vi "Begin.vi"(8 "error in":errorcluster) -> (0 "error out":errorcluster)   [LabVIEW 2023]
doc: "Called before other user functions, this VI can be used to open I/O refnums, load in file data, and do general program initialization. Notice that the <B>error out</B> terminal is simply used for data flow. Wiring it to other structures or subVIs ensures that this VI runs first."
uses:
  <vilib>/Rock Robotics/WPI/DriverStation/WPI_DriverStationRobotMode2.ctl
  <vilib>/Rock Robotics/WPI/Joystick/WPI_JoystickDeviceEnum.ctl
  Swerve/Implementation/Swerve Setpoints2.ctl
  Swerve/Implementation/Swerve Operations.ctl
  <vilib>/Rock Robotics/SystemInterfaces/DIO/FPGA_DIOChannel.ctl
  <vilib>/Rock Robotics/WPI/Solenoid/WPI_SolenoidChannel.ctl
  <vilib>/Rock Robotics/WPI/Solenoid/WPI_SolenoidValue.ctl
  <vilib>/Rock Robotics/WPI/SafetyOutput/WPI_SafetyOutputConfigMenu.ctl
  <vilib>/Rock Robotics/WPI/ThirdParty/REV Robotics/REVLib/Typedef/Spark MAX Idle Mode.ctl
  <vilib>/Rock Robotics/WPI/ThirdParty/REV Robotics/REVLib/Typedef/Spark MAX Sensor Type.ctl
  <vilib>/Rock Robotics/WPI/ThirdParty/REV Robotics/REVLib/Typedef/Spark MAX Control Type.ctl
  Robot Global Data.vi
  <vilib>/Rock Robotics/Network Tables/NT Write String Array.vi
  <vilib>/Rock Robotics/WPI/Solenoid/WPI_SolenoidOpenDouble.vi
  <vilib>/Rock Robotics/WPI/Solenoid/WPI_SolenoidSetEnum.vi
  <vilib>/Rock Robotics/WPI/Utilities/WPI_GetSetVariantRefNum.vi
  <vilib>/Rock Robotics/SystemInterfaces/DIO/FPGA_DIOPWMChannel.ctl
  Arm/Implementation/Arm Setpoints.ctl
panel:
  in  "Swerve PID":T1={"P Gain"=1.1, "I Gain"=0.0, "D Gain"=0.0, "F Gain"=0.0, "I Zone"=0.0, "Min Output"=-1.0, "Max Output"=1.0}
  in  "PID Constants 2":T1={"P Gain"=2.0, "I Gain"=0.0, "D Gain"=0.0, "F Gain"=0.0, "I Zone"=0.0, "Min Output"=-1.0, "Max Output"=1.0}
  in  "PID Constants":T1={"P Gain"=0.8, "I Gain"=0.0, "D Gain"=0.0, "F Gain"=0.0, "I Zone"=0.0, "Min Output"=-1.0, "Max Output"=1.0}
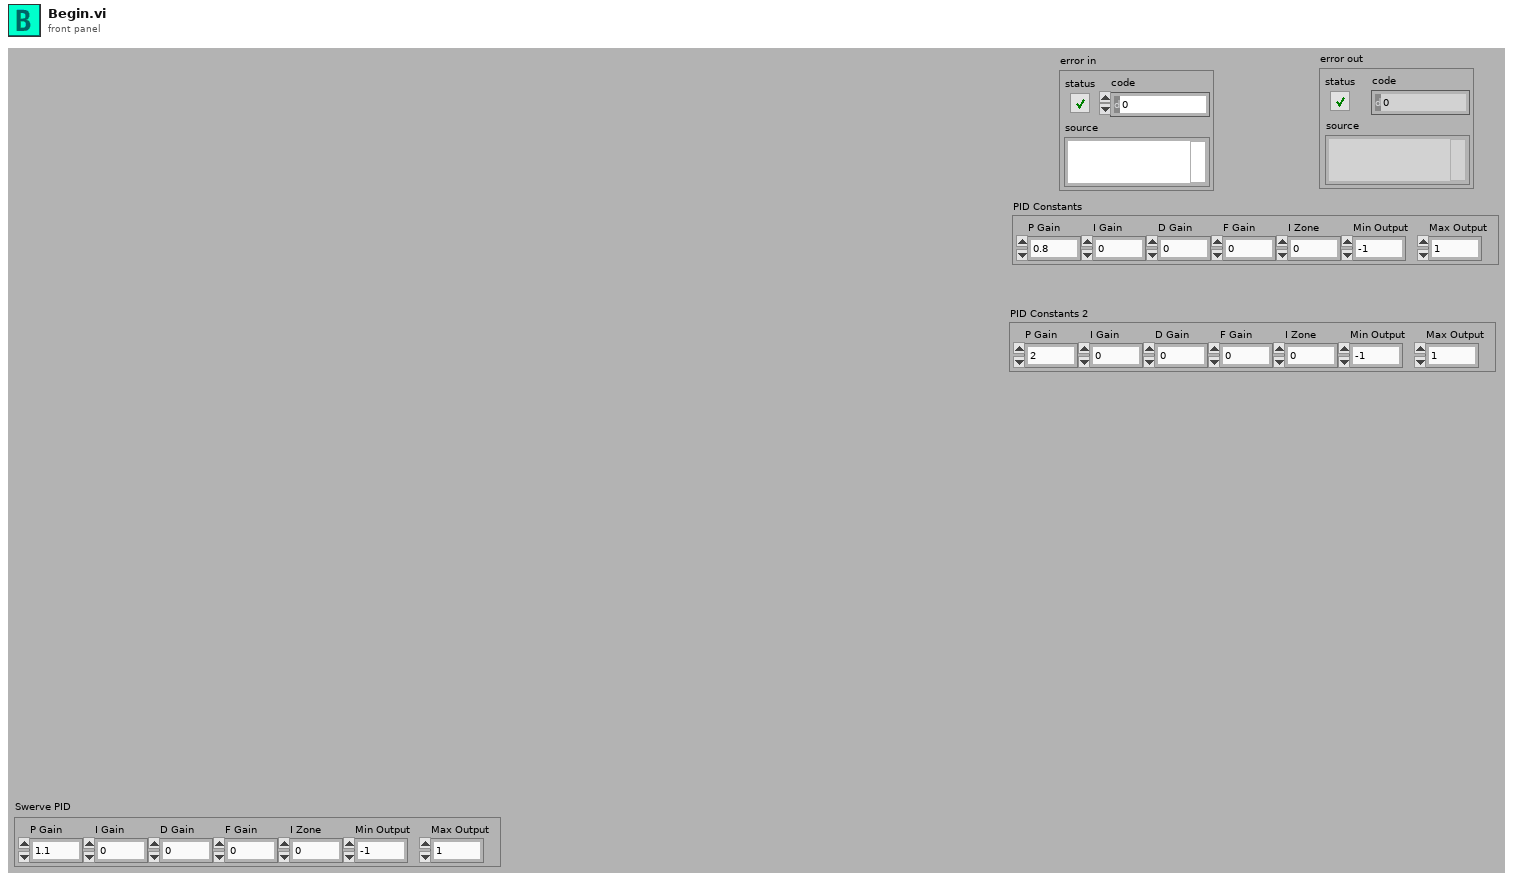
[diagram p1: front panel]
types:
  T1 = cluster{"P Gain":dbl, "I Gain":dbl, "D Gain":dbl, "F Gain":dbl, "I Zone":dbl, "Min Output":dbl, "Max Output":dbl}
  T2 = typedef "FPGA_DIOChannel.ctl" = enum8{"DIO 0", "DIO 1", "DIO 2", "DIO 3", "DIO 4", "DIO 5", "DIO 6", "DIO 7", "DIO 8", "DIO 9", "DIO MXP 0", "DIO MXP 1", "DIO MXP 2", "DIO MXP 3", "DIO MXP 4", "DIO MXP 5", "DIO MXP 6", "DIO MXP 7", "DIO MXP 8", "DIO MXP 9", "DIO MXP 10", "DIO MXP 11", "DIO MXP 12", "DIO MXP 13", "DIO MXP 14", "DIO MXP 15", "SPI Port CS1", "SPI Port CS2", "SPI Port CS3", "SPI Port MISO", "SPI Port MOSI", "Invalid"}
  T3 = typedef "Swerve Setpoints2.ctl" = cluster{"Operation":T4, "Gyro":dbl, "FWD":dbl, "STR":dbl, "X rotate":dbl, "Y rotate":dbl, "Time":dbl, "Distance":dbl, "Right Trigger":dbl, "Angle":dbl, "Start Angle":dbl, "Tag ID":dbl, "Start Positions":dbl[]}
  T4 = typedef "Swerve Operations.ctl" = enum16{"Reserve", "Read Current", "Immediate", "Stop", "Balance", "Direct  Joystick Drive", "Joystick Drive", "Drive for Distance", "Drive for Time", "Turn to Angle", "Drive to Angle(Time)", "Drive to Angle(Distance)", "Look At Cone", "Look At Cube", "Move To Tape", "Move To Tag"}
  T5 = typedef "WPI_JoystickDeviceEnum.ctl" = enum16{"USB 0", "USB 1", "USB 2", "USB 3", "USB 4", "USB 5"}
  T6 = typedef "WPI_DriverStationRobotMode2.ctl" = enum16{"Autonomous Disabled", "Autonomous Enabled", "Teleop Disabled", "Teleop Enabled", "Disconnected", "Finish", "Test Disabled", "Test Enabled", "Emergency Stopped"}
  T7 = typedef "Spark MAX Sensor Type.ctl" = enum16{"No Sensor", "Hall Sensor", "Encoder", "-Not Available-", "Analog", "Alternate Encoder", "Duty Cycle"}
  T8 = typedef "Spark MAX Idle Mode.ctl" = enum16{"Coast", "Brake"}
  T9 = typedef "WPI_SafetyOutputConfigMenu.ctl" = enum16{"Enable", "Disable"}
  T10 = typedef "WPI_MotorControlDeviceRef.ctl" = cluster{"DeviceStatus":errorcluster, "Type":T11, "PWM":cluster{"PWM Channel":T12, "DeadBand":T13}, "CAN":cluster{"Device Number":u8, "SetOutput VI Ref":variant, "GetOutput VI Ref":variant, "Enable VI Ref":variant, "Disable VI Ref":variant, "Data":variant}, "Invert":bool, "DIO PWM":cluster{"PWM \"Enable\" Channel":T12, "DIOChannel":T2, "PWM Rate":dbl}}
  T11 = typedef "WPI_MotorControlType.ctl" = enum16{"PWM", "CAN", "DIO PWM"}
  T12 = typedef "FPGA_DIOPWMChannel.ctl" = enum8{"PWM 0", "PWM 1", "PWM 2", "PWM 3", "PWM 4", "PWM 5", "PWM 6", "PWM 7", "PWM 8", "PWM 9", "PWM MXP 0", "PWM MXP 1", "PWM MXP 2", "PWM MXP 3", "PWM MXP 4", "PWM MXP 5", "PWM MXP 6", "PWM MXP 7", "PWM MXP 8", "PWM MXP 9", "Invalid"}
  T13 = typedef "WPI_PWMDeadband.ctl" = cluster{"Name":string, "maxPositivePwm":i32, "minPositivePwm":i32, "centerPwm":i32, "maxNegativePwm":i32, "minNegativePwm":i32, "angularRange":u16}
  T14 = typedef "WPI_JoystickDevRef.ctl" = cluster{"Device":T5}
  T15 = typedef "ADIS16470 Device Reference.ctl" = cluster{"DevStatus":errorcluster, "Hardware Config":T16, "Calibration Complete":refnum<notifier>, "Status Reference":refnum<data-value>, "Data Reference":refnum<data-value>, "Sychronous Process VI":T19, "Cmd FIFO":refnum<k33>, "Source":T20, "Data FIFO":refnum<k33>, "Calibration Time (ms)":u32, "Data Reference":refnum<data-value>}
  T16 = typedef "ADIS16470 Hardware Configuration.ctl" = cluster{"SPI Clock Rate (Hz)":dbl, "IMU SPI Mode (3)":T17, "IMU Reset Pin":T2, "IMU SPI Bus":T18, "IMU Data Ready Pin":T2, "Stall Config":cluster{"Pow2BytesPerRead":u8, "StallTicks":u16, "CsToSclkTicks":u8}}
  T17 = typedef "WPI_SPIMode.ctl" = enum16{"Mode 0 (Clk Idle Low,Sample on Leading)", "Mode 1 (Clk Idle Low,Sample on Trailing)", "Mode 2 (Clk Idle High,Sample on Leading)", "Mode 3 (Clk Idle High,Sample on Trailing)"}
  T18 = typedef "spi_bus.ctl" = enum16{"SPI On-Board, CS0", "SPI On-Board, CS1", "SPI On-Board, CS2", "SPI On-Board, CS3", "SPI MXP", "Invalid"}
  T19 = typedef "ADIS16470 Process.ctl" = refnum<vi>
  T20 = typedef "FPGA_CounterEncoderSourceConvertionLVSourceType.ctl" = cluster{"DevStatus":errorcluster, "AnalogTriggerMode?":bool, "DigitalMode":cluster{"DIO Channel":T21}, "AnalogTriggerMode":cluster{"AnalogTriggerIndex":T22, "OutputType":T23}}
  T21 = typedef "FPGA_DIODigitalSourceChannel.ctl" = enum8{"DIO 0", "DIO 1", "DIO 2", "DIO 3", "DIO 4", "DIO 5", "DIO 6", "DIO 7", "DIO 8", "DIO 9", "DIO MXP 0", "DIO MXP 1", "DIO MXP 2", "DIO MXP 3", "DIO MXP 4", "DIO MXP 5", "DIO MXP 6", "DIO MXP 7", "DIO MXP 8", "DIO MXP 9", "DIO MXP 10", "DIO MXP 11", "DIO MXP 12", "DIO MXP 13", "DIO MXP 14", "DIO MXP 15", "SPI Port CS1", "SPI Port CS2", "SPI Port CS3", "SPI Port MISO", "SPI Port MOSI", "Disabled"}
  T22 = typedef "FPGA_AnalogTriggerIndex.ctl" = enum8{"Trig 0", "Trig 1", "Trig 2", "Trig 3", "Trig 4", "Trig 5", "Trig 6", "Trig 7", "Invalid"}
  T23 = typedef "FPGA_AnalogTriggerOutType.ctl" = enum16{"InWindow", "TriggerState", "Rising", "Falling"}
  T24 = typedef "WPI_DigitalInputDevRef.ctl" = cluster{"DevStatus":errorcluster, "DIO Channel":T2}
  T25 = typedef "WPI_SolenoidValue.ctl" = enum16{"Off", "On", "Forward", "Reverse"}
  T26 = typedef "WPI_SolenoidChannel.ctl" = enum8{"Solenoid 0", "Solenoid 1", "Solenoid 2", "Solenoid 3", "Solenoid 4", "Solenoid 5", "Solenoid 6", "Solenoid 7", "Solenoid 8", "Solenoid 9", "Solenoid 10", "Solenoid 11", "Solenoid 12", "Solenoid 13", "Solenoid 14", "Solenoid 15", "Invalid"}
  T27 = typedef "WPI_CompressorDevRef.ctl" = cluster{"DevStatus":errorcluster, "Pneumatics Control Module":u8}
  T28 = typedef "WPI_SolenoidDevRef.ctl" = cluster{"DevStatus":errorcluster, "Pneumatics Control Module":u8, "Forward Solenoid Channel":T26, "Reverse Solenoid Channel":T26}
  T29 = typedef "WPI_PWMDeviceRef.ctl" = cluster{"DeviceStatus":errorcluster, "PWM Channel":T12}
  T30 = typedef "Spark MAX Control Type.ctl" = enum16{"Percent VBus", "Voltage", "Velocity", "Position", "Smart Motion", "Current", "Smart Velocity"}
  T31 = typedef "Arm Setpoints.ctl" = cluster{"Operation":enum16{"Reserve", "Read Current", "Immediate", "Move to position", "Adjust position", "Cube extend", "Cone extend", "Rotate Arm Joints", "Maintain Angle", "Retract", "Go_to_next"}, "X Position":dbl, "Y Position":dbl, "Up":dbl, "Right":dbl, "Joint 1 Angle":dbl[], "Joint 2 Angle":dbl[], "Joint 1 Speed":dbl, "Joint 2 Speed":dbl}
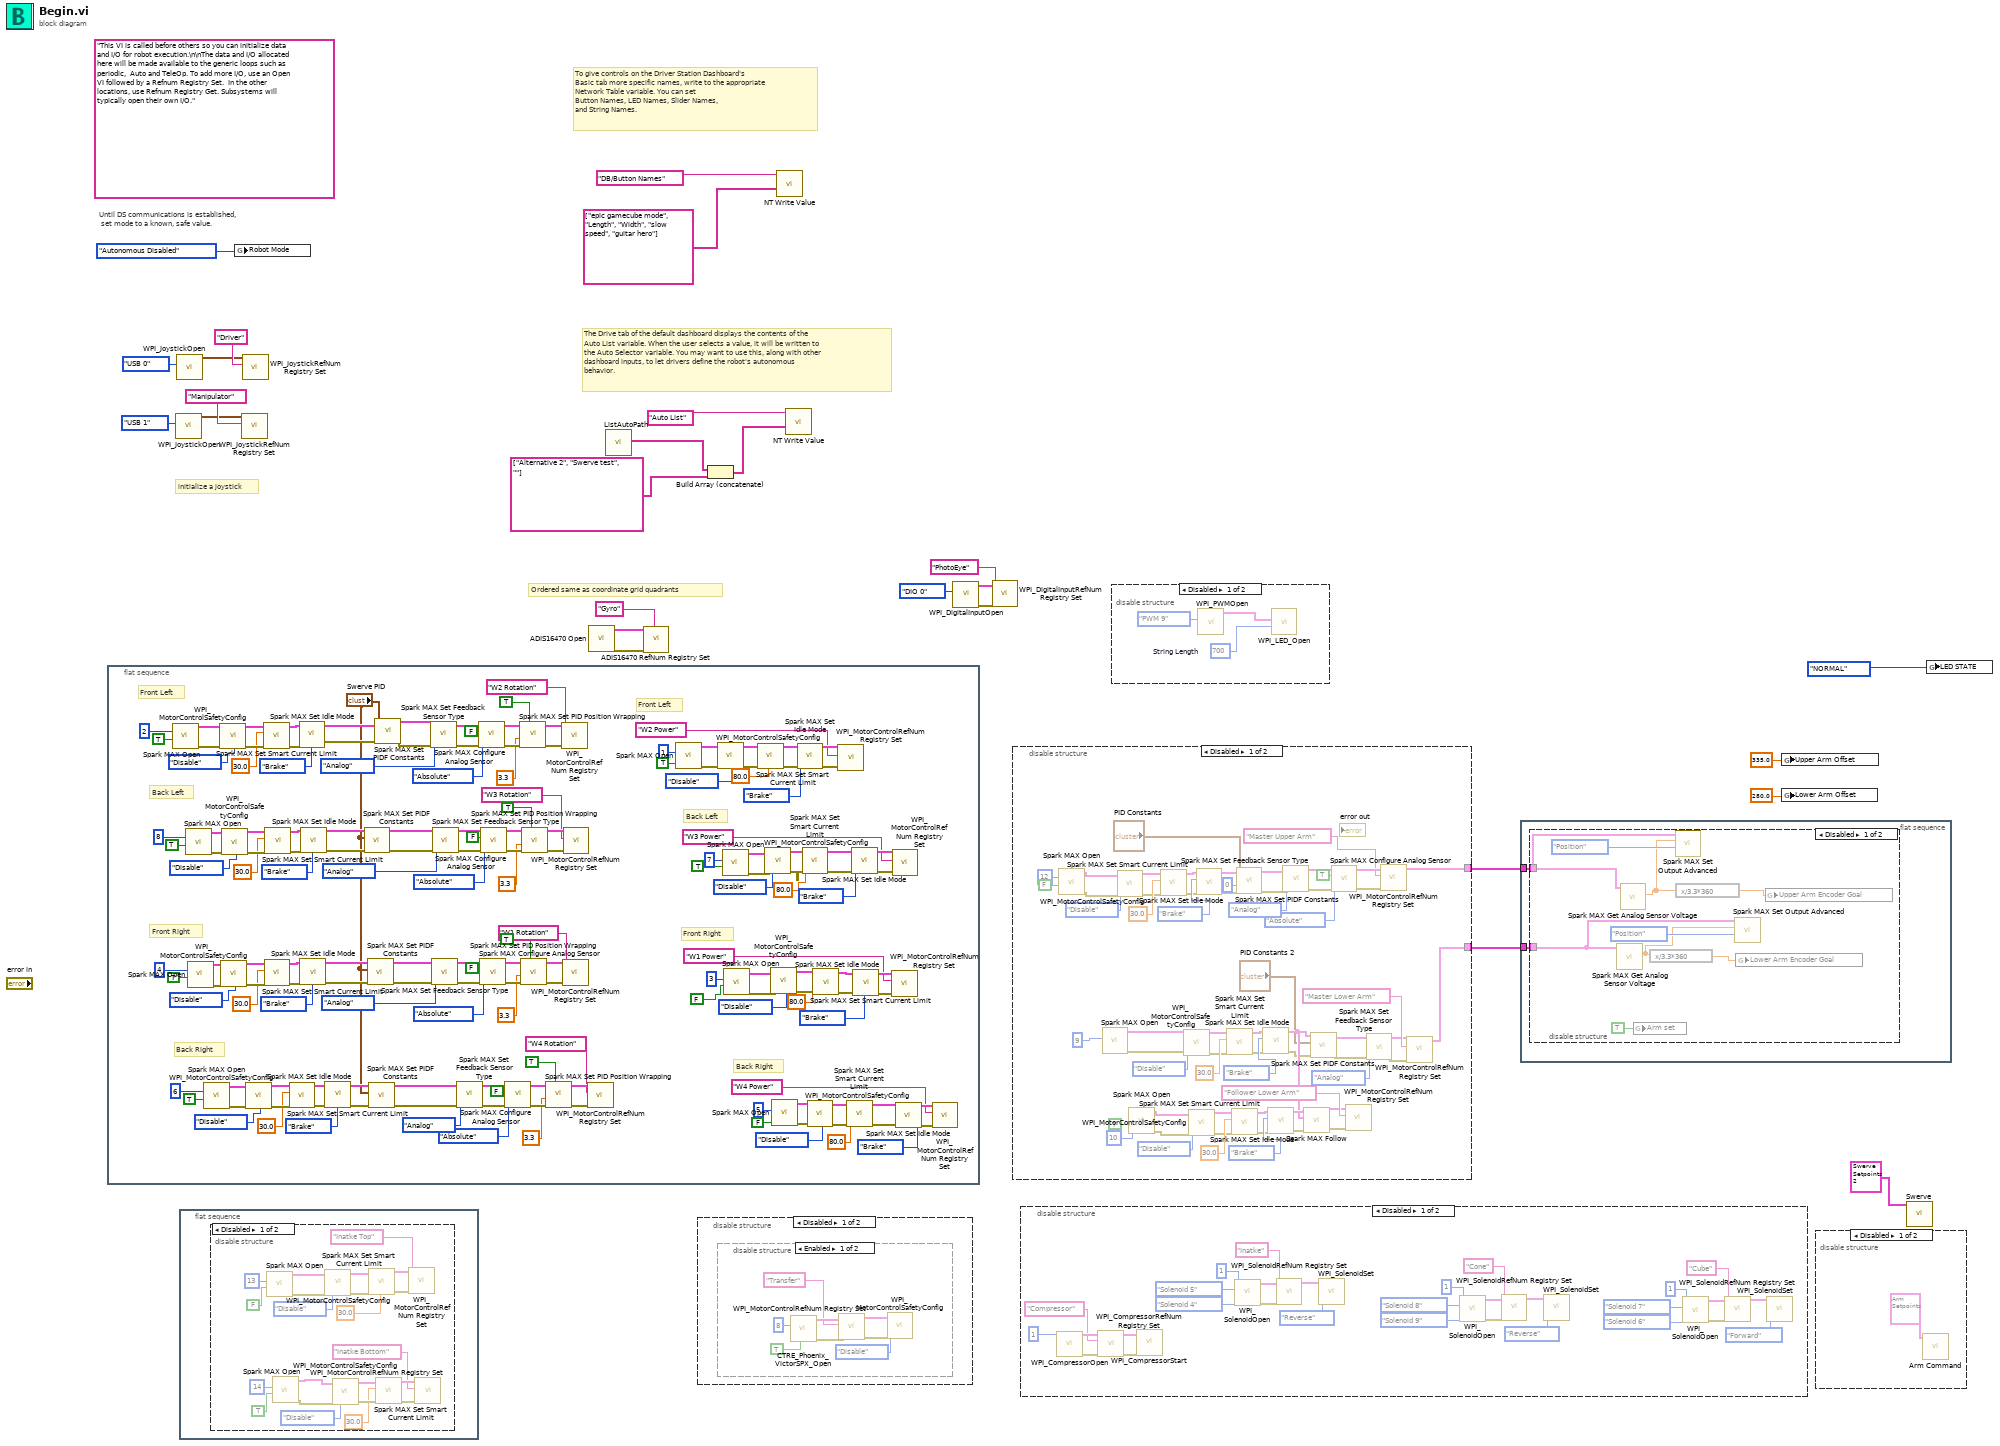
[diagram p0: block diagram]
diagram:
  (unwired) "This VI is called before others so you can initialize data and I/O for robot execution.\n\nThe data and I/O allocated here will be made available to the generic loops such as periodic,  Auto and TeleOp. To add more I/O, use an Open VI followed by a Refnum Registry Set.  In the other locations, use Refnum Registry Get. Subsystems will typically open their own I/O."
  # "Ordered same as coordinate grid quadrants"
  # "The Drive tab of the default dashboard displays the contents of the\nAuto List variable. When the user selects a value, it will be written to\nthe Auto Selector variable. You may want to use this, along with other\ndashboard inputs, to let drivers define the robot's autonomous\nbehavior."
  # "To give controls on the Driver Station Dashboard's\nBasic tab more specific names, write to the appropriate\nNetwork Table variable. You can set\nButton Names, LED Names, Slider Names,\nand String Names."
  # "initialize a joystick"
  # "Until DS communications is established,\n set mode to a known, safe value."
  n1 = flat-sequence {
    frame #0 {
      # "Back Right"
      # "Back Right"
      # "Front Right"
      # "Front Right"
      # "Back Left"
      # "Back Left"
      # "Front Left"
      # "Front Left"
      n2 = call <vilib>:"Spark MAX Open.vi"("Invert"=TRUE, "Device Number"=u8 2) -> ("error out"=w94:errorcluster, "MotorControlDeviceRef"=w95:T10)  [unwired: 8 in]
      n3 = call <vilib>:"Spark MAX Open.vi"("Invert"=TRUE, "Device Number"=u8 8) -> ("error out"=w164:errorcluster, "MotorControlDeviceRef"=w165:T10)  [unwired: 8 in]
      n4 = call <vilib>:"Spark MAX Open.vi"("Invert"=TRUE, "Device Number"=u8 4) -> ("error out"=w74:errorcluster, "MotorControlDeviceRef"=w75:T10)  [unwired: 8 in]
      n5 = call <vilib>:"Spark MAX Open.vi"("Invert"=TRUE, "Device Number"=u8 6) -> ("error out"=w54:errorcluster, "MotorControlDeviceRef"=w55:T10)  [unwired: 8 in]
      n6 = call <vilib>:"WPI_MotorControlSafetyConfig.vi"("error in (no error)"=w94, "mode"=WPI_SafetyOutputConfigMenu."Disable", "MotorControlDevRef"=w95) -> ("error out"=w112:errorcluster, "MotorControlDevRef"=w110:T10)  [unwired: 7 in]
      n7 = call <vilib>:"WPI_MotorControlSafetyConfig.vi"("error in (no error)"=w74, "mode"=WPI_SafetyOutputConfigMenu."Disable", "MotorControlDevRef"=w75) -> ("error out"=w92:errorcluster, "MotorControlDevRef"=w90:T10)  [unwired: 7 in]
      n8 = call <vilib>:"WPI_MotorControlSafetyConfig.vi"("error in (no error)"=w164, "mode"=WPI_SafetyOutputConfigMenu."Disable", "MotorControlDevRef"=w165) -> ("error out"=w175:errorcluster, "MotorControlDevRef"=w168:T10)  [unwired: 7 in]
      n9 = call <vilib>:"WPI_MotorControlSafetyConfig.vi"("error in (no error)"=w54, "mode"=WPI_SafetyOutputConfigMenu."Disable", "MotorControlDevRef"=w55) -> ("error out"=w72:errorcluster, "MotorControlDevRef"=w70:T10)  [unwired: 7 in]
      n10 = call <vilib>:"Spark MAX Set Smart Current Limit.vi"("error in (no error)"=w112, "Primay Current Limit (80A)"=30.0, "MotorControlDeviceRef in"=w110) -> ("error out"=w113:errorcluster, "MotorControlDeviceRef out"=w111:T10)  [unwired: 7 in]
      n11 = call <vilib>:"Spark MAX Set Smart Current Limit.vi"("error in (no error)"=w92, "Primay Current Limit (80A)"=30.0, "MotorControlDeviceRef in"=w90) -> ("error out"=w93:errorcluster, "MotorControlDeviceRef out"=w91:T10)  [unwired: 7 in]
      n12 = call <vilib>:"Spark MAX Set Smart Current Limit.vi"("error in (no error)"=w175, "Primay Current Limit (80A)"=30.0, "MotorControlDeviceRef in"=w168) -> ("error out"=w176:errorcluster, "MotorControlDeviceRef out"=w172:T10)  [unwired: 7 in]
      n13 = call <vilib>:"Spark MAX Set Smart Current Limit.vi"("error in (no error)"=w72, "Primay Current Limit (80A)"=30.0, "MotorControlDeviceRef in"=w70) -> ("error out"=w73:errorcluster, "MotorControlDeviceRef out"=w71:T10)  [unwired: 7 in]
      n14 = call <vilib>:"Spark MAX Set Idle Mode.vi"("error in (no error)"=w113, "Idle Mode"=Spark_MAX_Idle_Mode."Brake", "MotorControlDeviceRef in"=w111) -> ("error out"=w45:errorcluster, "MotorControlDeviceRef out"=w44:T10)  [unwired: 7 in]
      n15 = call <vilib>:"Spark MAX Set Idle Mode.vi"("error in (no error)"=w93, "Idle Mode"=Spark_MAX_Idle_Mode."Brake", "MotorControlDeviceRef in"=w91) -> ("error out"=w37:errorcluster, "MotorControlDeviceRef out"=w38:T10)  [unwired: 7 in]
      n16 = call <vilib>:"Spark MAX Set Idle Mode.vi"("error in (no error)"=w176, "Idle Mode"=Spark_MAX_Idle_Mode."Brake", "MotorControlDeviceRef in"=w172) -> ("error out"=w41:errorcluster, "MotorControlDeviceRef out"=w42:T10)  [unwired: 7 in]
      n17 = call <vilib>:"Spark MAX Set Idle Mode.vi"("error in (no error)"=w73, "Idle Mode"=Spark_MAX_Idle_Mode."Brake", "MotorControlDeviceRef in"=w71) -> ("error out"=w33:errorcluster, "MotorControlDeviceRef out"=w34:T10)  [unwired: 7 in]
      n18 = call <vilib>:"Spark MAX Set PIDF Constants.vi"("error in"=w41, "PID Constants"="Swerve PID", "MotorControlDeviceRef"=w42) -> ("error out"=w39:errorcluster, "MotorControlDeviceRef"=w40:T10)  [unwired: 7 in]
      n19 = call <vilib>:"Spark MAX Set PIDF Constants.vi"("error in"=w37, "PID Constants"="Swerve PID", "MotorControlDeviceRef"=w38) -> ("error out"=w35:errorcluster, "MotorControlDeviceRef"=w36:T10)  [unwired: 7 in]
      n20 = call <vilib>:"Spark MAX Set PIDF Constants.vi"("error in"=w33, "PID Constants"="Swerve PID", "MotorControlDeviceRef"=w34) -> ("error out"=w31:errorcluster, "MotorControlDeviceRef"=w32:T10)  [unwired: 7 in]
      n21 = call <vilib>:"Spark MAX Set PIDF Constants.vi"("error in"=w45, "PID Constants"="Swerve PID", "MotorControlDeviceRef"=w44) -> ("error out"=w46:errorcluster, "MotorControlDeviceRef"=w47:T10)  [unwired: 7 in]
      n22 = call <vilib>:"Spark MAX Set Feedback Sensor Type.vi"("error in (no error)"=w46, "Sensor Type"=Spark_MAX_Sensor_Type."Analog", "MotorControlDevRef"=w47) -> ("error out"=w103:errorcluster, "MotorControlDeviceRef"=w104:T10)  [unwired: 7 in]
      n23 = call <vilib>:"Spark MAX Set Feedback Sensor Type.vi"("error in (no error)"=w35, "Sensor Type"=Spark_MAX_Sensor_Type."Analog", "MotorControlDevRef"=w36) -> ("error out"=w83:errorcluster, "MotorControlDeviceRef"=w84:T10)  [unwired: 7 in]
      n24 = call <vilib>:"Spark MAX Set Feedback Sensor Type.vi"("error in (no error)"=w39, "Sensor Type"=Spark_MAX_Sensor_Type."Analog", "MotorControlDevRef"=w40) -> ("error out"=w122:errorcluster, "MotorControlDeviceRef"=w123:T10)  [unwired: 7 in]
      n25 = call <vilib>:"Spark MAX Set Feedback Sensor Type.vi"("error in (no error)"=w31, "Sensor Type"=Spark_MAX_Sensor_Type."Analog", "MotorControlDevRef"=w32) -> ("error out"=w63:errorcluster, "MotorControlDeviceRef"=w64:T10)  [unwired: 7 in]
      n26 = call <vilib>:"Spark MAX Configure Analog Sensor.vi"("error in (no error)"=w103, "Sensor Mode (Absolute)"=enum16{"Absolute", "Relative"}."Absolute", "Inverted (F)"=FALSE, "MotorControlDeviceRef in"=w104) -> ("error out"=w100:errorcluster, "MotorControlDeviceRef"=w101:T10)  [unwired: 6 in]
      n27 = call <vilib>:"Spark MAX Configure Analog Sensor.vi"("error in (no error)"=w83, "Sensor Mode (Absolute)"=enum16{"Absolute", "Relative"}."Absolute", "Inverted (F)"=FALSE, "MotorControlDeviceRef in"=w84) -> ("error out"=w80:errorcluster, "MotorControlDeviceRef"=w81:T10)  [unwired: 6 in]
      n28 = call <vilib>:"Spark MAX Configure Analog Sensor.vi"("error in (no error)"=w122, "Sensor Mode (Absolute)"=enum16{"Absolute", "Relative"}."Absolute", "Inverted (F)"=FALSE, "MotorControlDeviceRef in"=w123) -> ("error out"=w119:errorcluster, "MotorControlDeviceRef"=w120:T10)  [unwired: 6 in]
      n29 = call <vilib>:"Spark MAX Configure Analog Sensor.vi"("error in (no error)"=w63, "Sensor Mode (Absolute)"=enum16{"Absolute", "Relative"}."Absolute", "Inverted (F)"=FALSE, "MotorControlDeviceRef in"=w64) -> ("error out"=w60:errorcluster, "MotorControlDeviceRef"=w61:T10)  [unwired: 6 in]
      n30 = call <vilib>:"Spark MAX Set PID Position Wrapping.vi"("Enable (F)"=TRUE, "error in (no error)"=w100, "Maximum Output (0)"=3.3, "MotorControlDeviceRef in"=w101) -> ("error out"=w99:errorcluster, "MotorControlDeviceRef out"=w98:T10)  [unwired: 6 in]
      n31 = call <vilib>:"Spark MAX Set PID Position Wrapping.vi"("Enable (F)"=TRUE, "error in (no error)"=w80, "Maximum Output (0)"=3.3, "MotorControlDeviceRef in"=w81) -> ("error out"=w79:errorcluster, "MotorControlDeviceRef out"=w78:T10)  [unwired: 6 in]
      n32 = call <vilib>:"Spark MAX Set PID Position Wrapping.vi"("Enable (F)"=TRUE, "error in (no error)"=w119, "Maximum Output (0)"=3.3, "MotorControlDeviceRef in"=w120) -> ("error out"=w118:errorcluster, "MotorControlDeviceRef out"=w117:T10)  [unwired: 6 in]
      n33 = call <vilib>:"Spark MAX Set PID Position Wrapping.vi"("Enable (F)"=TRUE, "error in (no error)"=w60, "Maximum Output (0)"=3.3, "MotorControlDeviceRef in"=w61) -> ("error out"=w59:errorcluster, "MotorControlDeviceRef out"=w58:T10)  [unwired: 6 in]
      n34 = call <vilib>:"WPI_MotorControlRefNum Registry Set.vi"("error in (no error)"=w99, "refnum name"="W2 Rotation", "MotorControlDevRef"=w98) -> ()  [unwired: 7 in, 2 out]
      n35 = call <vilib>:"WPI_MotorControlRefNum Registry Set.vi"("error in (no error)"=w79, "refnum name"="W1 Rotation", "MotorControlDevRef"=w78) -> ()  [unwired: 7 in, 2 out]
      n36 = call <vilib>:"WPI_MotorControlRefNum Registry Set.vi"("error in (no error)"=w118, "refnum name"="W3 Rotation", "MotorControlDevRef"=w117) -> ()  [unwired: 7 in, 2 out]
      n37 = call <vilib>:"WPI_MotorControlRefNum Registry Set.vi"("error in (no error)"=w59, "refnum name"="W4 Rotation", "MotorControlDevRef"=w58) -> ()  [unwired: 7 in, 2 out]
      n38 = call <vilib>:"Spark MAX Open.vi"("Invert"=TRUE, "Device Number"=u8 1) -> ("error out"=w184:errorcluster, "MotorControlDeviceRef"=w185:T10)  [unwired: 8 in]
      n39 = call <vilib>:"WPI_MotorControlSafetyConfig.vi"("error in (no error)"=w184, "mode"=WPI_SafetyOutputConfigMenu."Disable", "MotorControlDevRef"=w185) -> ("error out"=w186:errorcluster, "MotorControlDevRef"=w187:T10)  [unwired: 7 in]
      n40 = call <vilib>:"Spark MAX Open.vi"("Invert"=TRUE, "Device Number"=u8 7) -> ("error out"=w166:errorcluster, "MotorControlDeviceRef"=w167:T10)  [unwired: 8 in]
      n41 = call <vilib>:"Spark MAX Open.vi"("Invert"=FALSE, "Device Number"=u8 3) -> ("error out"=w147:errorcluster, "MotorControlDeviceRef"=w148:T10)  [unwired: 8 in]
      n42 = call <vilib>:"Spark MAX Set Smart Current Limit.vi"("error in (no error)"=w186, "Primay Current Limit (80A)"=80.0, "MotorControlDeviceRef in"=w187) -> ("error out"=w188:errorcluster, "MotorControlDeviceRef out"=w189:T10)  [unwired: 7 in]
      n43 = call <vilib>:"WPI_MotorControlSafetyConfig.vi"("error in (no error)"=w166, "mode"=WPI_SafetyOutputConfigMenu."Disable", "MotorControlDevRef"=w167) -> ("error out"=w177:errorcluster, "MotorControlDevRef"=w169:T10)  [unwired: 7 in]
      n44 = call <vilib>:"WPI_MotorControlSafetyConfig.vi"("error in (no error)"=w147, "mode"=WPI_SafetyOutputConfigMenu."Disable", "MotorControlDevRef"=w148) -> ("error out"=w149:errorcluster, "MotorControlDevRef"=w150:T10)  [unwired: 7 in]
      n45 = call <vilib>:"Spark MAX Open.vi"("Invert"=FALSE, "Device Number"=u8 5) -> ("error out"=w132:errorcluster, "MotorControlDeviceRef"=w133:T10)  [unwired: 8 in]
      n46 = call <vilib>:"Spark MAX Set Idle Mode.vi"("error in (no error)"=w188, "Idle Mode"=Spark_MAX_Idle_Mode."Brake", "MotorControlDeviceRef in"=w189) -> ("error out"=w190:errorcluster, "MotorControlDeviceRef out"=w191:T10)  [unwired: 7 in]
      n47 = call <vilib>:"Spark MAX Set Smart Current Limit.vi"("error in (no error)"=w177, "Primay Current Limit (80A)"=80.0, "MotorControlDeviceRef in"=w169) -> ("error out"=w170:errorcluster, "MotorControlDeviceRef out"=w171:T10)  [unwired: 7 in]
      n48 = call <vilib>:"WPI_MotorControlSafetyConfig.vi"("error in (no error)"=w132, "mode"=WPI_SafetyOutputConfigMenu."Disable", "MotorControlDevRef"=w133) -> ("error out"=w134:errorcluster, "MotorControlDevRef"=w135:T10)  [unwired: 7 in]
      n49 = call <vilib>:"Spark MAX Set Smart Current Limit.vi"("error in (no error)"=w149, "Primay Current Limit (80A)"=80.0, "MotorControlDeviceRef in"=w150) -> ("error out"=w154:errorcluster, "MotorControlDeviceRef out"=w151:T10)  [unwired: 7 in]
      n50 = call <vilib>:"WPI_MotorControlRefNum Registry Set.vi"("error in (no error)"=w190, "refnum name"="W2 Power", "MotorControlDevRef"=w191) -> ()  [unwired: 7 in, 2 out]
      n51 = call <vilib>:"Spark MAX Set Smart Current Limit.vi"("error in (no error)"=w134, "Primay Current Limit (80A)"=80.0, "MotorControlDeviceRef in"=w135) -> ("error out"=w136:errorcluster, "MotorControlDeviceRef out"=w137:T10)  [unwired: 7 in]
      n52 = call <vilib>:"Spark MAX Set Idle Mode.vi"("error in (no error)"=w170, "Idle Mode"=Spark_MAX_Idle_Mode."Brake", "MotorControlDeviceRef in"=w171) -> ("error out"=w174:errorcluster, "MotorControlDeviceRef out"=w173:T10)  [unwired: 7 in]
      n53 = call <vilib>:"Spark MAX Set Idle Mode.vi"("error in (no error)"=w154, "Idle Mode"=Spark_MAX_Idle_Mode."Brake", "MotorControlDeviceRef in"=w151) -> ("error out"=w152:errorcluster, "MotorControlDeviceRef out"=w153:T10)  [unwired: 7 in]
      n54 = call <vilib>:"WPI_MotorControlRefNum Registry Set.vi"("error in (no error)"=w152, "refnum name"="W1 Power", "MotorControlDevRef"=w153) -> ()  [unwired: 7 in, 2 out]
      n55 = call <vilib>:"WPI_MotorControlRefNum Registry Set.vi"("error in (no error)"=w174, "refnum name"="W3 Power", "MotorControlDevRef"=w173) -> ()  [unwired: 7 in, 2 out]
      n56 = call <vilib>:"Spark MAX Set Idle Mode.vi"("error in (no error)"=w136, "Idle Mode"=Spark_MAX_Idle_Mode."Brake", "MotorControlDeviceRef in"=w137) -> ("error out"=w138:errorcluster, "MotorControlDeviceRef out"=w139:T10)  [unwired: 7 in]
      n57 = call <vilib>:"WPI_MotorControlRefNum Registry Set.vi"("error in (no error)"=w138, "refnum name"="W4 Power", "MotorControlDevRef"=w139) -> ()  [unwired: 7 in, 2 out]
    }
  }
  n58 = call <vilib>:"WPI_JoystickOpen.vi"("JoystickDevice"=WPI_JoystickDeviceEnum."USB 1") -> ("JoystickDevRef"=w18:T14)  [unwired: 10 in]
  n59 = call <vilib>:"WPI_JoystickOpen.vi"("JoystickDevice"=WPI_JoystickDeviceEnum."USB 0") -> ("JoystickDevRef"=w24:T14)  [unwired: 10 in]
  n60 = flat-sequence {
    frame #0 {
      n61 = disable-structure shown="Disabled" {
        frame Disabled {
          n62 = call <vilib>:"Spark MAX Open.vi"("Invert"=FALSE, "Device Number"=u8 13) -> ("error out"=w207:errorcluster, "MotorControlDeviceRef"=w206:T10)  [unwired: 8 in]
          n63 = call <vilib>:"Spark MAX Open.vi"("Invert"=TRUE, "Device Number"=u8 14) -> ("error out"=w212:errorcluster, "MotorControlDeviceRef"=w211:T10)  [unwired: 8 in]
          n64 = call <vilib>:"WPI_MotorControlSafetyConfig.vi"("error in (no error)"=w207, "mode"=WPI_SafetyOutputConfigMenu."Disable", "MotorControlDevRef"=w206) -> ("error out"=w213:errorcluster, "MotorControlDevRef"=w202:T10)  [unwired: 7 in]
          n65 = call <vilib>:"WPI_MotorControlSafetyConfig.vi"("error in (no error)"=w212, "mode"=WPI_SafetyOutputConfigMenu."Disable", "MotorControlDevRef"=w211) -> ("error out"=w210:errorcluster, "MotorControlDevRef"=w203:T10)  [unwired: 7 in]
          n66 = call <vilib>:"Spark MAX Set Smart Current Limit.vi"("error in (no error)"=w213, "Primay Current Limit (80A)"=30.0, "MotorControlDeviceRef in"=w202) -> ("error out"=w205:errorcluster, "MotorControlDeviceRef out"=w204:T10)  [unwired: 7 in]
          n67 = call <vilib>:"Spark MAX Set Smart Current Limit.vi"("error in (no error)"=w210, "Primay Current Limit (80A)"=30.0, "MotorControlDeviceRef in"=w203) -> ("error out"=w209:errorcluster, "MotorControlDeviceRef out"=w208:T10)  [unwired: 7 in]
          n68 = call <vilib>:"WPI_MotorControlRefNum Registry Set.vi"("error in (no error)"=w205, "refnum name"="Inatke Top", "MotorControlDevRef"=w204) -> ()  [unwired: 7 in, 2 out]
          n69 = call <vilib>:"WPI_MotorControlRefNum Registry Set.vi"("error in (no error)"=w209, "refnum name"="Inatke Bottom", "MotorControlDevRef"=w208) -> ()  [unwired: 7 in, 2 out]
        }
        frame Enabled {
        }
      }
    }
  }
  n70 = global write "Robot Global Data.vi" "Robot Mode"(WPI_DriverStationRobotMode2."Autonomous Disabled" ("Robot Mode")) -> ()
  n71 = call <vilib>:"WPI_JoystickRefNum Registry Set.vi"("refnum name"="Manipulator", "JoystickDevRef"=w18) -> ()  [unwired: 8 in, 2 out]
  n72 = call <vilib>:"WPI_JoystickRefNum Registry Set.vi"("refnum name"="Driver", "JoystickDevRef"=w24) -> ()  [unwired: 8 in, 2 out]
  n73 = call <vilib>:"ADIS16470 Open.vi"() -> ("error out"=w1:errorcluster, "ADIS16470DevRef"=w13:T15)  [unwired: 10 in]
  n74 = call "ListAutoPath.vi"() -> ("AutoRoutinesNames"=w15:string[])  [unwired: 11 in]
  n75 = call <vilib>:"ADIS16470 RefNum Registry Set.vi"("error in (no error)"=w1, "refnum name"="Gyro", "ADIS16470DevRef in"=w13) -> ()  [unwired: 7 in, 2 out]
  n76 = disable-structure shown="Disabled" {
    frame Disabled {
      n77 = disable-structure shown="Enabled" {
        frame Enabled {
          n78 = call <vilib>:"CTRE_Phoenix_VictorSPX_Open.vi"("Invert"=TRUE, "Device Number"=u8 8) -> ("error out"=w215:errorcluster, "PhoenixMotorControlDevRef"=w217:T10)  [unwired: 8 in]
          n79 = call <vilib>:"WPI_MotorControlRefNum Registry Set.vi"("error in (no error)"=w215, "refnum name"="Transfer", "MotorControlDevRef"=w217) -> ("error out"=w220:errorcluster, "MotorControlDevRef"=w219:T10)  [unwired: 7 in]
          n80 = call <vilib>:"WPI_MotorControlSafetyConfig.vi"("error in (no error)"=w220, "mode"=WPI_SafetyOutputConfigMenu."Disable", "MotorControlDevRef"=w219) -> ()  [unwired: 7 in, 2 out]
        }
        frame Disabled {
        }
      }
    }
    frame Enabled {
    }
  }
  n81 = Build Array (concatenate)(w15, string[] ["Alternative 2", "Swerve test", ""] ("String Array")) -> (w16:string[])
  n82 = call-poly <vilib>:"NT Write Value.vi"("value"=string[] ["epic gamecube mode", "Length", "Width", "slow speed", "guitar hero"] ("String Array"), "name"="DB/Button Names" ("Name")) -> ()  [unwired: 9 in, 1 out]
  n83 = call-poly <vilib>:"NT Write Value.vi"("value"=w16, "name"="Auto List" ("Name")) -> ()  [unwired: 9 in, 1 out]
  n84 = call <vilib>:"WPI_DigitalInputOpen.vi"("DIO Channel"=FPGA_DIOChannel."DIO 0") -> ("error out"=w9:errorcluster, "DigitalInputDevRef"=w8:T24)  [unwired: 9 in]
  n85 = call <vilib>:"WPI_DigitalInputRefNum Registry Set.vi"("error in (no error)"=w9, "refnum name"="PhotoEye", "DigitalInputDevRef"=w8) -> ()  [unwired: 7 in, 2 out]
  n86 = disable-structure shown="Disabled" {
    disable-tunnel: [w223 _] -> w4
    disable-tunnel: [w222 _] -> w3
    frame Disabled {
      n87 = call <vilib>:"Spark MAX Open.vi"("Invert"=FALSE, "Device Number"=u8 12) -> ("error out"=w240:errorcluster, "MotorControlDeviceRef"=w241:T10)  [unwired: 8 in]
      n88 = call <vilib>:"Spark MAX Open.vi"("Device Number"=u8 9) -> ("error out"=w247:errorcluster, "MotorControlDeviceRef"=w248:T10)  [unwired: 9 in]
      n89 = call <vilib>:"WPI_MotorControlSafetyConfig.vi"("error in (no error)"=w240, "mode"=WPI_SafetyOutputConfigMenu."Disable", "MotorControlDevRef"=w241) -> ("error out"=w239:errorcluster, "MotorControlDevRef"=w282:T10)  [unwired: 7 in]
      n90 = call <vilib>:"Spark MAX Open.vi"("Invert"=TRUE, "Device Number"=u8 10) -> ("error out"=w242:errorcluster, "MotorControlDeviceRef"=w243:T10)  [unwired: 8 in]
      n91 = call <vilib>:"Spark MAX Set Smart Current Limit.vi"("error in (no error)"=w239, "Primay Current Limit (80A)"=30.0, "MotorControlDeviceRef in"=w282) -> ("error out"=w238:errorcluster, "MotorControlDeviceRef out"=w279:T10)  [unwired: 7 in]
      n92 = call <vilib>:"WPI_MotorControlSafetyConfig.vi"("error in (no error)"=w247, "mode"=WPI_SafetyOutputConfigMenu."Disable", "MotorControlDevRef"=w248) -> ("error out"=w237:errorcluster, "MotorControlDevRef"=w271:T10)  [unwired: 7 in]
      n93 = call <vilib>:"WPI_MotorControlSafetyConfig.vi"("error in (no error)"=w242, "mode"=WPI_SafetyOutputConfigMenu."Disable", "MotorControlDevRef"=w243) -> ("error out"=w234:errorcluster, "MotorControlDevRef"=w277:T10)  [unwired: 7 in]
      n94 = call <vilib>:"Spark MAX Set Idle Mode.vi"("error in (no error)"=w238, "Idle Mode"=Spark_MAX_Idle_Mode."Brake", "MotorControlDeviceRef in"=w279) -> ("error out"=w262:errorcluster, "MotorControlDeviceRef out"=w261:T10)  [unwired: 7 in]
      n95 = call <vilib>:"Spark MAX Set Smart Current Limit.vi"("error in (no error)"=w237, "Primay Current Limit (80A)"=30.0, "MotorControlDeviceRef in"=w271) -> ("error out"=w236:errorcluster, "MotorControlDeviceRef out"=w268:T10)  [unwired: 7 in]
      n96 = call <vilib>:"Spark MAX Set Smart Current Limit.vi"("error in (no error)"=w234, "Primay Current Limit (80A)"=30.0, "MotorControlDeviceRef in"=w277) -> ("error out"=w233:errorcluster, "MotorControlDeviceRef out"=w274:T10)  [unwired: 7 in]
      n97 = call <vilib>:"Spark MAX Set PIDF Constants.vi"("error in"=w262, "PIDF Slot"=0, "PID Constants"="PID Constants", "MotorControlDeviceRef"=w261) -> ("error out"=w257:errorcluster, "MotorControlDeviceRef"=w256:T10)  [unwired: 6 in]
      n98 = call <vilib>:"Spark MAX Set Idle Mode.vi"("error in (no error)"=w236, "Idle Mode"=Spark_MAX_Idle_Mode."Brake", "MotorControlDeviceRef in"=w268) -> ("error out"=w235:errorcluster, "MotorControlDeviceRef out"=w259:T10)  [unwired: 7 in]
      n99 = call <vilib>:"Spark MAX Set Idle Mode.vi"("error in (no error)"=w233, "Idle Mode"=Spark_MAX_Idle_Mode."Brake", "MotorControlDeviceRef in"=w274) -> ("error out"=w232:errorcluster, "MotorControlDeviceRef out"=w273:T10)  [unwired: 7 in]
      n100 = call <vilib>:"Spark MAX Set Feedback Sensor Type.vi"("error in (no error)"=w257, "Sensor Type"=Spark_MAX_Sensor_Type."Analog", "MotorControlDevRef"=w256) -> ("error out"=w229:errorcluster, "MotorControlDeviceRef"=w230:T10)  [unwired: 7 in]
      n101 = call <vilib>:"Spark MAX Follow.vi"("error in (no error)"=w232, "Master Controller"=w259, "MotorControlDeviceRef"=w273) -> ("error out"=w244:errorcluster, "MotorControlDeviceRef"=w245:T10)  [unwired: 7 in]
      n102 = call <vilib>:"Spark MAX Set PIDF Constants.vi"("error in"=w235, "PID Constants"="PID Constants 2", "MotorControlDeviceRef"=w259) -> ("error out"=w252:errorcluster, "MotorControlDeviceRef"=w253:T10)  [unwired: 7 in]
      n103 = call <vilib>:"Spark MAX Configure Analog Sensor.vi"("error in (no error)"=w229, "Sensor Mode (Absolute)"=enum16{"Absolute", "Relative"}."Absolute", "Inverted (F)"=TRUE, "MotorControlDeviceRef in"=w230) -> ("error out"=w226:errorcluster, "MotorControlDeviceRef"=w227:T10)  [unwired: 6 in]
      n104 = call <vilib>:"WPI_MotorControlRefNum Registry Set.vi"("error in (no error)"=w244, "refnum name"="Follower Lower Arm", "MotorControlDevRef"=w245) -> ()  [unwired: 7 in, 2 out]
      n105 = call <vilib>:"Spark MAX Set Feedback Sensor Type.vi"("error in (no error)"=w252, "Sensor Type"=Spark_MAX_Sensor_Type."Analog", "MotorControlDevRef"=w253) -> ("error out"=w249:errorcluster, "MotorControlDeviceRef"=w250:T10)  [unwired: 7 in]
      n106 = call <vilib>:"WPI_MotorControlRefNum Registry Set.vi"("error in (no error)"=w226, "refnum name"="Master Upper Arm", "MotorControlDevRef"=w227) -> ("MotorControlDevRef"=w223:T10)  [unwired: 7 in, 1 out]
      n107 = call <vilib>:"WPI_MotorControlRefNum Registry Set.vi"("error in (no error)"=w249, "refnum name"="Master Lower Arm", "MotorControlDevRef"=w250) -> ("MotorControlDevRef"=w222:T10)  [unwired: 7 in, 1 out]
    }
    frame Enabled {
    }
  }
  n108 = disable-structure shown="Disabled" {
    frame Disabled {
      n109 = call <vilib>:"WPI_CompressorOpen.vi"("Pneumatics device (def)"=u8 1) -> ("CompressorDevRef"=w288:T27, "error out"=w289:errorcluster)  [unwired: 13 in]
      n110 = call <vilib>:"WPI_CompressorRefNum Registry Set.vi"("error in (no error)"=w289, "refnum name"="Compressor", "CompressorDevRef"=w288) -> ("error out"=w287:errorcluster, "CompressorDevRef"=w286:T27)  [unwired: 7 in]
      n111 = call <vilib>:"WPI_CompressorStart.vi"("error in (no error)"=w287, "CompressorDevRef"=w286) -> ()  [unwired: 8 in, 2 out]
      n112 = call-poly <vilib>:"WPI_SolenoidOpen.vi"("Reverse Solenoid Channel"=WPI_SolenoidChannel."Solenoid 4", "Forward Solenoid Channel"=WPI_SolenoidChannel."Solenoid 5", "Pneumatics Device (def)"=u8 1) -> ("error out"=w310:errorcluster, "SolenoidDevRef"=w309:T28)  [unwired: 7 in]
      n113 = call <vilib>:"WPI_SolenoidRefNum Registry Set.vi"("error in (no error)"=w310, "refnum name"="Inatke", "SolenoidDevRef"=w309) -> ("SolenoidDevRef"=w306:T28)  [unwired: 7 in, 1 out]
      n114 = call-poly <vilib>:"WPI_SolenoidSet.vi"("Value"=WPI_SolenoidValue."Reverse", "SolenoidDevRef"=w306) -> ()  [unwired: 8 in, 2 out]
      n115 = call-poly <vilib>:"WPI_SolenoidOpen.vi"("Reverse Solenoid Channel"=WPI_SolenoidChannel."Solenoid 9", "Forward Solenoid Channel"=WPI_SolenoidChannel."Solenoid 8", "Pneumatics Device (def)"=u8 1) -> ("error out"=w302:errorcluster, "SolenoidDevRef"=w301:T28)  [unwired: 7 in]
      n116 = call <vilib>:"WPI_SolenoidRefNum Registry Set.vi"("error in (no error)"=w302, "refnum name"="Cone", "SolenoidDevRef"=w301) -> ("SolenoidDevRef"=w298:T28)  [unwired: 7 in, 1 out]
      n117 = call-poly <vilib>:"WPI_SolenoidSet.vi"("Value"=WPI_SolenoidValue."Reverse", "SolenoidDevRef"=w298) -> ()  [unwired: 8 in, 2 out]
      n118 = call-poly <vilib>:"WPI_SolenoidOpen.vi"("Reverse Solenoid Channel"=WPI_SolenoidChannel."Solenoid 6", "Forward Solenoid Channel"=WPI_SolenoidChannel."Solenoid 7", "Pneumatics Device (def)"=u8 1) -> ("error out"=w294:errorcluster, "SolenoidDevRef"=w293:T28)  [unwired: 7 in]
      n119 = call <vilib>:"WPI_SolenoidRefNum Registry Set.vi"("error in (no error)"=w294, "refnum name"="Cube", "SolenoidDevRef"=w293) -> ("SolenoidDevRef"=w290:T28)  [unwired: 7 in, 1 out]
      n120 = call-poly <vilib>:"WPI_SolenoidSet.vi"("Value"=WPI_SolenoidValue."Forward", "SolenoidDevRef"=w290) -> ()  [unwired: 8 in, 2 out]
    }
    frame Enabled {
    }
  }
  n121 = disable-structure shown="Disabled" {
    frame Disabled {
      w314 = u16 700  # String Length
      n122 = call <vilib>:"WPI_PWMOpen.vi"("PWM Channel"=FPGA_DIOPWMChannel."PWM 9") -> ("PWMDeviceRef"=w316:T29)  [unwired: 9 in, 1 out]
      n123 = call <vilib>:"WPI_LED_Open.vi"("String Length"=w314, "PWMDeviceRef"=w316) -> ()  [unwired: 9 in, 1 out]
    }
    frame Enabled {
    }
  }
  n124 = flat-sequence {
    tunnel: w4 -> [w318]
    tunnel: w3 -> [w317]
    frame #0 {
      n125 = disable-structure shown="Disabled" {
        disable-tunnel: w318 -> [w323 _]
        disable-tunnel: w317 -> [w320 _]
        frame Disabled {
          n126 = call <vilib>:"Spark MAX Get Analog Sensor Voltage.vi"("MotorControlDevRef in"=w320) -> ("Analog Sensor Voltage"=w319:dbl)  [unwired: 7 in, 3 out]
          n127 = call <vilib>:"Spark MAX Get Analog Sensor Voltage.vi"("MotorControlDevRef in"=w323) -> ("Analog Sensor Voltage"=w322:dbl)  [unwired: 7 in, 3 out]
          n128 = global write "Robot Global Data.vi" "Arm set"(TRUE ("Arm set")) -> ()
          n129 = expression code="x/3.3*360"(w319) -> (w327:dbl)
          n130 = call <vilib>:"Spark MAX Set Output Advanced.vi"("Control Mode"=Spark_MAX_Control_Type."Position", "Setpoint"=w322, "MotorControlDevRef"=w323) -> ()  [unwired: 7 in, 2 out]
          n131 = expression code="x/3.3*360"(w322) -> (w326:dbl)
          n132 = call <vilib>:"Spark MAX Set Output Advanced.vi"("Control Mode"=Spark_MAX_Control_Type."Position", "Setpoint"=w319, "MotorControlDevRef"=w320) -> ()  [unwired: 7 in, 2 out]
          n133 = global write "Robot Global Data.vi" "Lower Arm Encoder Goal"(w327) -> ()
          n134 = global write "Robot Global Data.vi" "Upper Arm Encoder Goal"(w326) -> ()
        }
        frame Enabled {
        }
      }
    }
  }
  n135 = global write "Robot Global Data.vi" "Upper Arm Offset"(335.0 ("Upper Arm Offset")) -> ()
  n136 = global write "Robot Global Data.vi" "Lower Arm Offset"(280.0 ("Upper Arm Offset")) -> ()
  n137 = disable-structure shown="Disabled" {
    frame Disabled {
      n138 = call "Arm Command.vi"("SubSystem Data"=T31 {"Operation"=enum."Rotate Arm Joints", "X Position"=0.0, "Y Position"=0.0, "Up"=0.0, "Right"=0.0, "Joint 1 Angle"=[], "Joint 2 Angle"=[], "Joint 1 Speed"=0.0, "Joint 2 Speed"=0.0}) -> ()  [unwired: 10 in, 1 out]
    }
    frame Enabled {
    }
  }
  n139 = call "Swerve.vi"("SubSystem Data"=T3 {"Operation"=enum."Joystick Drive", "Gyro"=0.0, "FWD"=0.0, "STR"=0.0, "X rotate"=0.0, "Y rotate"=0.0, "Time"=0.0, "Distance"=0.0, "Right Trigger"=0.0, "Angle"=0.0, "Start Angle"=0.0, "Tag ID"=0.0, "Start Positions"=[]}) -> ()  [unwired: 10 in, 1 out]
  n140 = global write "Robot Global Data.vi" "LED STATE"(enum16{"NORMAL", "RAINBOW"}."NORMAL" ("LED STATE")) -> ()
